vi "Example Authenticate - Connected Callback.vi"(4 "Connected":refnum<user-event>, 5 "Event Data":T1, 6 "Control Ref":refnum<k24>, 7 "Event Common Data":T2) -> ()   [LabVIEW 2010]
uses:
  C:/tf/play/labview/Tinkerforge.dll
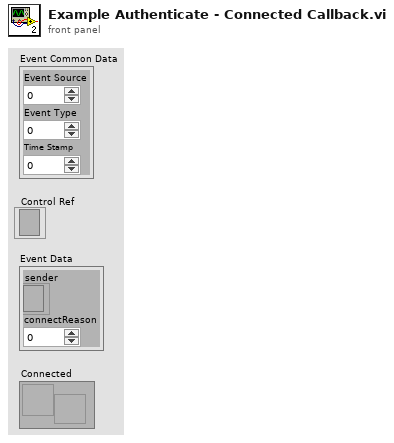
[diagram p1: front panel]
types:
  T1 = cluster{"sender":refnum<k24>, "connectReason":i16}
  T2 = cluster{"Event Source":i32, "Event Type":u32, "Time Stamp":u32}
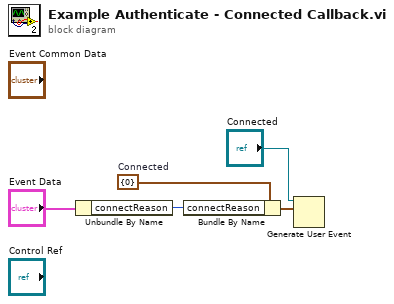
[diagram p0: block diagram]
diagram:
  w4 = cluster{"connectReason":i16} {"connectReason"=0}  # Connected
  n1 = Unbundle By Name("Event Data") -> ("connectReason"=w3:i16)
  n2 = Bundle By Name(cluster=w4, "connectReason"=w3) -> (w2:cluster{"connectReason":i16})
  n3 = Generate User Event(user event="Connected", event data cluster=w2) -> ()  [unwired: 1 in, 2 out]
